vi "Set Variant.vi"(8 "error in (no error)":errorcluster, 10 "Variant":variant, 11 "int32 in":refnum<class "string.lvclass">) -> (0 "error out":errorcluster, 3 "int32 out":refnum<class "string.lvclass">)   [LabVIEW 2020]
uses:
  string.lvclass
  string.lvclass/string.ctl
  E:/Labview/LV 2020/Libs/LV Protobuf Raw/Source/Proto Type Common/Proto Type Common.lvclass
  E:/Labview/LV 2020/Libs/LV Protobuf Raw/Source/Tag/Basic Type.lvclass
  E:/Labview/LV 2020/Libs/LV Protobuf Raw/Source/Proto Value/Proto Type.lvclass
  E:/Labview/LV 2020/Libs/LV Protobuf Raw/Source/Type Serializer/Type Serializer.lvclass
  E:/Labview/LV 2020/Libs/LV Protobuf Raw/Source/String Representable/String Representable.lvclass
  E:/Labview/LV 2020/Libs/LV Protobuf Raw/Source/Wire Type Group/Wire Type Group.lvclass
  E:/Labview/LV 2020/Libs/LV Protobuf Raw/Source/LEN Encoder/LEN.lvclass
  E:/Labview/LV 2020/Libs/LV Protobuf Raw/Source/string/string.lvclass
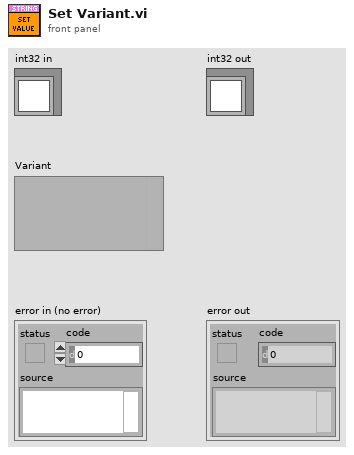
[diagram p1: front panel]
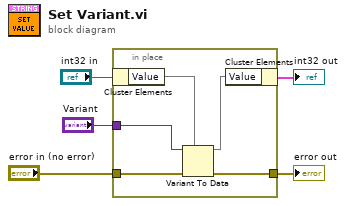
[diagram p0: block diagram]
diagram:
  n1 = in-place {
    in-place-border: "error in (no error)" -> [w10]
    in-place-border: [w9] -> w2
    in-place-border: "Variant" -> [w8]
    n2 = in-place-cluster #1("int32 in") -> ("Value"=w7)
    n3 = Variant To Data(error in=w10, type=w7, Variant=w8) -> (data=w6, error out=w9:errorcluster)
    n4 = in-place-cluster #1("Value"=w6) -> (→"int32 out":cluster{})
  }
  "error out" <- w2
